vi "Display and Record.vi"(0 "Tension (g)":dbl, 1 "t < 1.5 s ?":bool, 2 "Frequency (Hz)":dbl, 3 "User List":string[](array[string]), 5 "dT (g)":dbl, 7 "Wire Length (mm)":dbl, 9 "Linear Density (µm/mm)":dbl, 11 "Nth Measurement":i32, 12 "User ID":i32, 13 "sMDT Code":string) -> (4 "Data Array":string[][](array[string]), 6 "Frequency Out":dbl, 8 "Tension Out":dbl, 10 "dT Out":dbl, 14 "Linear Density Out":dbl, 15 "Wire Length Out":dbl)   [LabVIEW 2018]
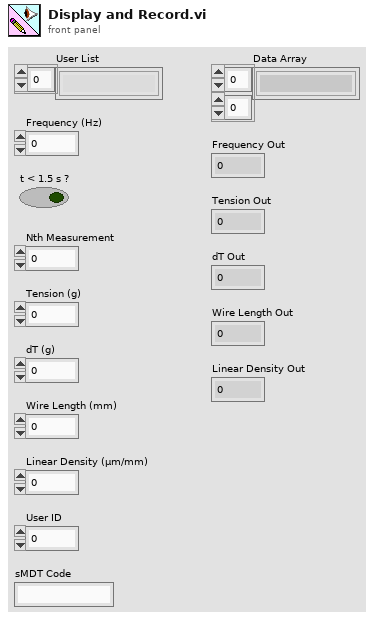
[diagram p1: front panel]
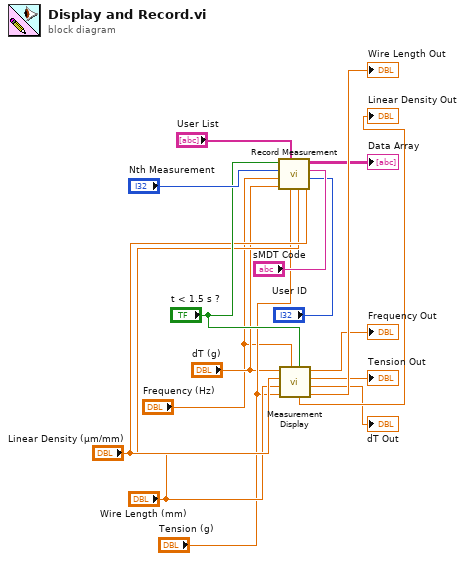
[diagram p0: block diagram]
diagram:
  n1 = call "Record Measurement.vi"("Linear Density"="Linear Density (µm/mm)", "Operator ID"="User ID", "sMDT Code"="sMDT Code", "Wire Length"="Wire Length (mm)", "Tension"="Tension (g)", "User List"="User List", "Uncertainty"="dT (g)", "Frequency"="Frequency (Hz)", "Nth measurement"="Nth Measurement", "t < X ?"="t < 1.5 s ?") -> ("Measurements"=→"Data Array":string[][])  [unwired: 1 in]
  n2 = call "Measurement Display.vi"("Boolean"="t < 1.5 s ?", "Frequency In"="Frequency (Hz)", "Tension In"="Tension (g)", "Wire Length In"="Wire Length (mm)", "Linear Density In"="Linear Density (µm/mm)", "dT In"="dT (g)") -> ("Wire Length Out"=→"Wire Length Out":dbl, "dT Out"=→"dT Out":dbl, "Tension Out"=→"Tension Out":dbl, "Frequency Out"=→"Frequency Out":dbl, "Linear Density Out"=→"Linear Density Out":dbl)  [unwired: 1 in]
